vi "PH_TKTDS-30xx.ProcEvents.vi"(0 "i ref in":refnum<vi>, 5 "error in":errorcluster) -> (14 "i ref out":refnum<vi>, 19 "error out":errorcluster)   [LabVIEW 2014, in "PH_TKTDS-30xx.lvlib"]
doc: "This method is used to define the events the object will listen to. Add your own events here."
uses:
  PH_TKTDS-30xx.lvlib
  CSCore/BaseProcess/BaseProcess.event definition.ctl
  CSCore/CAEObj/CAEObj.event definition.ctl
  CSCore/BaseProcess/BaseProcess.descriptor string definition.ctl
  CSCore/BaseProcess/BaseProcess.lvlib
  CSCore/CAEObj/CAEObj.lvlib
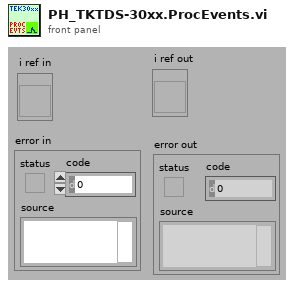
[diagram p1: front panel]
types:
  T1 = typedef "BaseProcess.lvlib/BaseProcess.event definition.ctl" = cluster{"CAEEvtDef":T2, "Data Descriptor":T3}
  T2 = typedef "CAEObj.lvlib/CAEObj.event definition.ctl" = cluster{"URL":string, "enable":bool, "ignoreResID":bool}
  T3 = typedef "BaseProcess.lvlib/BaseProcess.descriptor string definition.ctl" = string
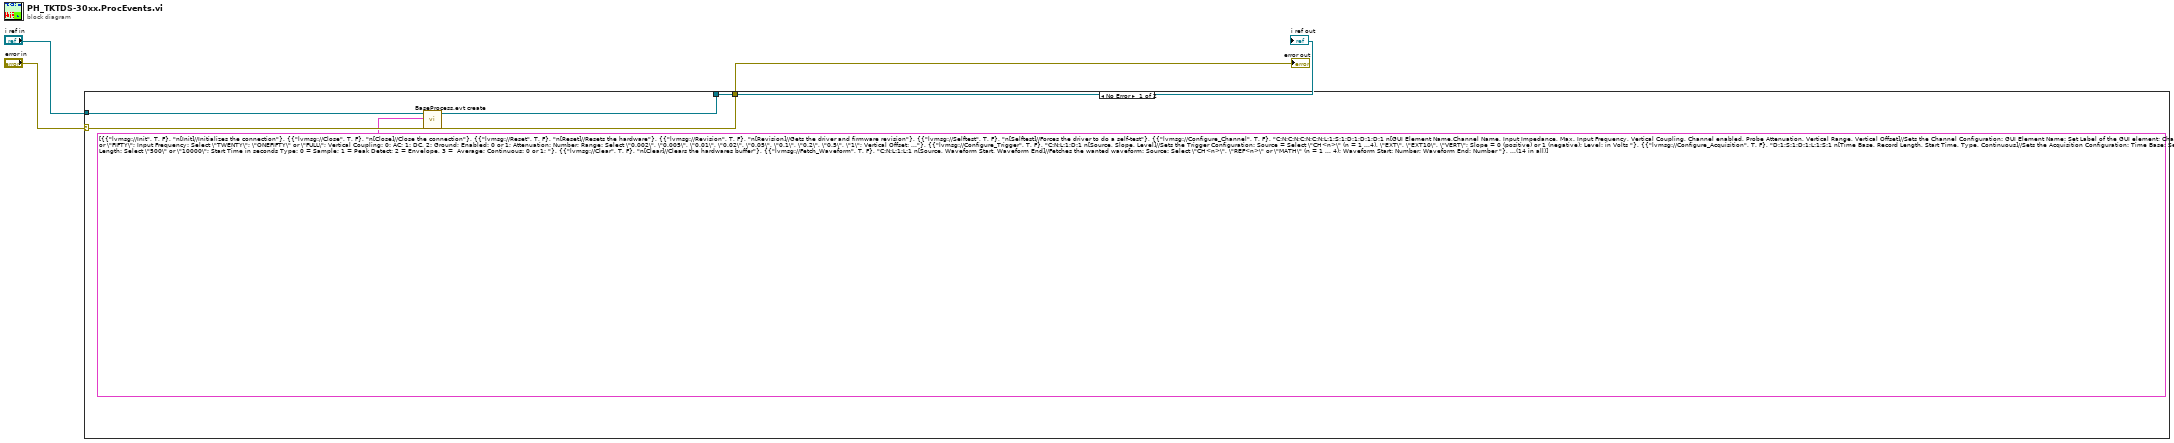
[diagram p0: block diagram]
diagram:
  n1 = case shown="No Error" "error in" {
    selector: "error in" -> [w7 w10]
    tunnel: "i ref in" -> [w6 w11]
    tunnel: [w9 w11] -> w3
    tunnel: [w8 w10] -> w2
    frame No Error {
      n2 = call "BaseProcess.evt create.vi"("i ref in"=w6, "newEvents"=T1[] [{"CAEEvtDef"={"URL"="lvmsg://Init", "enable"=TRUE, "ignoreResID"=FALSE}, "Data Descriptor"="n[Init]//Initializes the connection"}, {"CAEEvtDef"={"URL"="lvmsg://Close", "enable"=TRUE, "ignoreResID"=FALSE}, "Data Descriptor"="n[Close]//Close the connection"}, {"CAEEvtDef"={"URL"="lvmsg://Reset", "enable"=TRUE, "ignoreResID"=FALSE}, "Data Descriptor"="n[Reset]//Resets the hardware"}, {"CAEEvtDef"={"URL"="lvmsg://Revision", "enable"=TRUE, "ignoreResID"=FALSE}, "Data Descriptor"="n[Revision]//Gets the driver and firmware revision"}, {"CAEEvtDef"={"URL"="lvmsg://Selftest", "enable"=TRUE, "ignoreResID"=FALSE}, "Data Descriptor"="n[Selftest]//Forces the driver to do a self-test"}, {"CAEEvtDef"={"URL"="lvmsg://Configure_Channel", "enable"=TRUE, "ignoreResID"=FALSE}, "Data Descriptor"="C:N;C:N;C:N;C:N;L:1;S:1;D:1;D:1;D:1 n[GUI Element Name,Channel Name, Input Impedance, Max. Input Frequency, Vertical Coupling, Channel enabled, Probe Attenuation, Vertical Range, Vertical Offset]//Sets the Channel Configuration: GUI Element Name: Set Label of the GUI element; Channel Name: Select \"CH<n>\" (n = 1 ...4);  Input Impedance: Select \"MEG\" or \"FIFTY\"; Input Frequency: Select \"TWENTY\"; \"ONEFIFTY\" or \"FULL\"; Vertical Coupling: 0: AC; 1: DC, 2: Ground; Enabled: 0 or 1; Attenuation: Number; Range: Select \"0.002\", \"0.005\", \"0.01\", \"0.02\", \"0.05\", \"0.1\", \"0.2\", \"0.5\", \"1\"; Vertical Offset: Number "}, {"CAEEvtDef"={"URL"="lvmsg://Configure_Trigger", "enable"=TRUE, "ignoreResID"=FALSE}, "Data Descriptor"="C:N;L:1;D:1 n[Source, Slope, Level]//Sets the Trigger Configuration: Source = Select \"CH<n>\" (n = 1 ...4), \"EXT\", \"EXT10\", \"VERT\"; Slope = 0 (positive) or 1 (negative); Level: in Volts "}, {"CAEEvtDef"={"URL"="lvmsg://Configure_Acquisition", "enable"=TRUE, "ignoreResID"=FALSE}, "Data Descriptor"="D:1;S:1;D:1;L:1;S:1 n[Time Base, Record Length, Start Time, Type, Continuous]//Sets the Acquisition Configuration: Time Base: Select \"2E-9\", \"4E-9\", \"1E-8\", \"2E-8\", \"4E-8\", ... \"1\", \"2\", \"4\" or \"10\"; Record Length: Select \"500\" or \"10000\"; Start Time in seconds Type: 0 = Sample; 1 = Peak Detect; 2 = Envelope, 3 =  Average; Continuous: 0 or 1; "}, {"CAEEvtDef"={"URL"="lvmsg://Clear", "enable"=TRUE, "ignoreResID"=FALSE}, "Data Descriptor"="n[Clear]//Clears the hardwares buffer"}, {"CAEEvtDef"={"URL"="lvmsg://Fetch_Waveform", "enable"=TRUE, "ignoreResID"=FALSE}, "Data Descriptor"="C:N;L:1;L:1 n[Source, Waveform Start, Waveform End]//Fetches the wanted waveform: Source: Select \"CH<n>\", \"REF<n>\" or \"MATH\" (n = 1 ... 4); Waveform Start: Number; Waveform End: Number "}, {"CAEEvtDef"={"URL"="lvmsg://Set_Bin_Data_Encoding", "enable"=TRUE, "ignoreResID"=FALSE}, "Data Descriptor"="n[Bin data Encoding]//Set the hardware to a certain mode"}, {"CAEEvtDef"={"URL"="lvmsg://Remote Control", "enable"=TRUE, "ignoreResID"=FALSE}, "Data Descriptor"="S:1 n[Remote Control]//Sets the instance to be remotely controlled"}, {"CAEEvtDef"={"URL"="lvmsg://Set_Channel_Position", "enable"=TRUE, "ignoreResID"=FALSE}, "Data Descriptor"="C:N;D:1 n[Channel, Postion]//Sets the position of the specified channel in divisions of the display"}, {"CAEEvtDef"={"URL"="lvmsg://Set_Display_Intensity", "enable"=TRUE, "ignoreResID"=FALSE}, "Data Descriptor"="S:1 n[Display Intensity]//Sets the display intensity"}] ("new events"), "error in (no error)"=w7) -> ("i ref out"=w9:refnum<vi>, "error out"=w8:errorcluster)  [unwired: 13 in, 2 out]
    }
    frame Error {
    }
  }
  "i ref out" <- w3
  "error out" <- w2
